vi "RDV-init.vi"(8 "error in (no error)":errorcluster, 11 "RDV-Reflection_Data_viewer in":refnum<class "RDV-Reflection_Data_viewer.lvclass">) -> (0 "error out":errorcluster, 3 "RDV-Reflection_Data_viewer out":refnum<class "RDV-Reflection_Data_viewer.lvclass">)   [LabVIEW 2020, in "RDV-Reflection_Data_viewer.lvclass"]
uses:
  RDV-Reflection_Data_viewer.lvclass
  RDV-Reflection_Data_viewer.lvclass/RDV-Reflection_Data_viewer.ctl
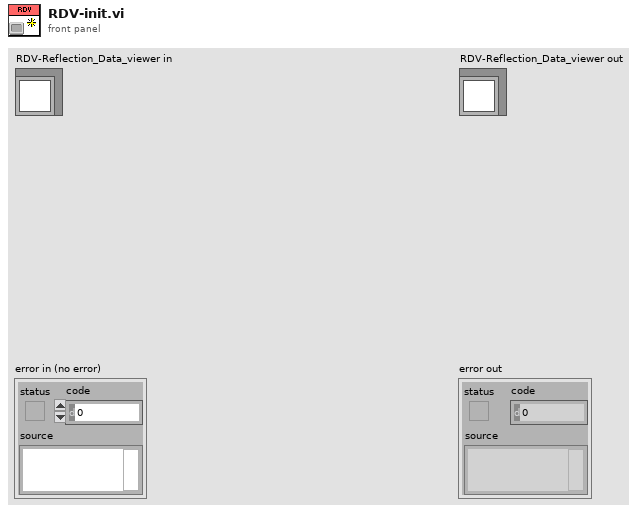
[diagram p1: front panel]
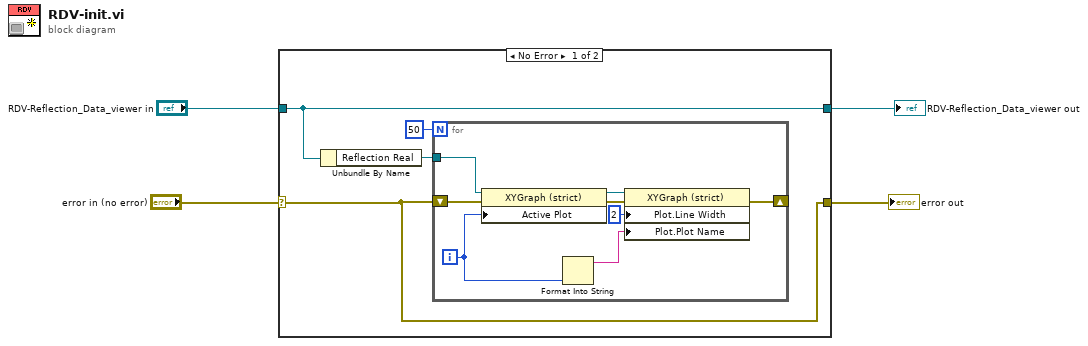
[diagram p0: block diagram]
diagram:
  n1 = case shown="No Error" "error in (no error)" {
    selector: "error in (no error)" -> [w5 w18]
    tunnel: [w5 w18] -> w3
    tunnel: [w8 w17] -> w1
    tunnel: "RDV-Reflection_Data_viewer in" -> [w8 w17]
    frame No Error {
      n2 = Unbundle By Name(w8) -> ("Reflection Real"=w7:refnum<vi>)
      n3 = for {
        N: 50 -> [_]
        tunnel: w7 -> [w12]
        shift-right: [w9] -> _
        shift-left: w5 -> [w11]
        i -> [w13]
        n4 = property on="Property Node" class="XYGraph (strict)"(reference=w12, error in=w11, "Active Plot"=w13) -> (reference out=w15:refnum<vi>, error out=w16:errorcluster)
        n5 = Format Into String(w13) -> (resulting string=w10:string)  [unwired: 3 in, 1 out]
        n6 = property on="Property Node" class="XYGraph (strict)"(reference=w15, error in=w16, "Plot.Line Width"=u8 2, "Plot.Plot Name"=w10) -> (error out=w9:errorcluster)  [unwired: 1 out]
      }
    }
    frame Error {
    }
  }
  "error out" <- w3
  "RDV-Reflection_Data_viewer out" <- w1
